vi "Phasor Weber 2-component Calculation.vi"(0 "Phasor 1 (g, s)":T1, 5 "Harmonic Order 1":i32, 7 "Phasor 2 (g, s)":T1, 9 "Harmonic Order 2":i32, 11 "Error In":errorcluster) -> (4 "Reduced Lifetime 1":dbl, 6 "Fraction 1":dbl, 8 "Reduced Lifetime 2":dbl, 10 "Fraction 2":dbl, 15 "Error Out":errorcluster)   [LabVIEW 2021, in "Phasor.lvlib"]
uses:
  Phasor (g, s).ctl
  Phasor.lvlib
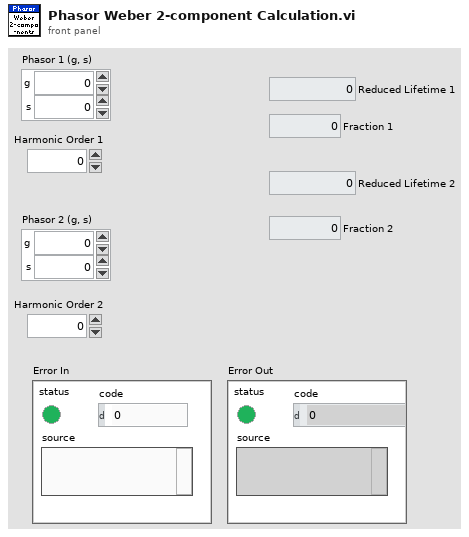
[diagram p1: front panel]
types:
  T1 = typedef "Phasor.lvlib/Phasor (g, s).ctl" = cluster{"g":dbl, "s":dbl}
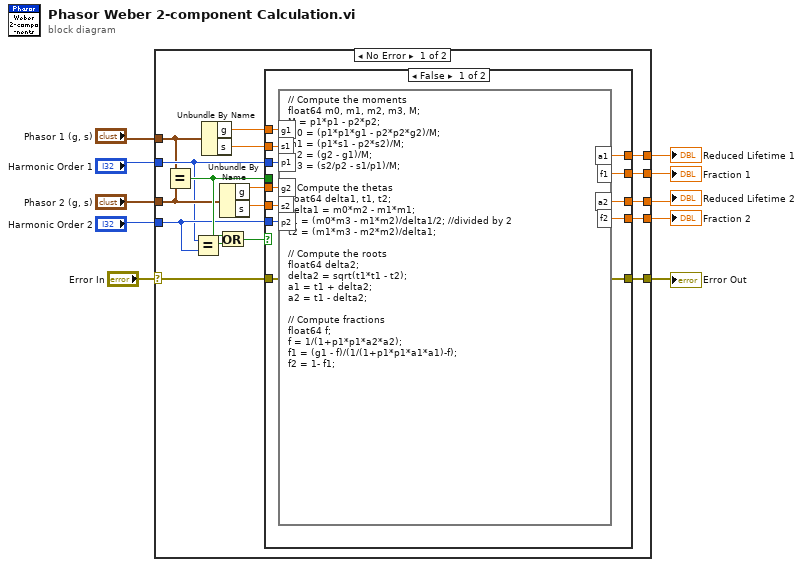
[diagram p0: block diagram]
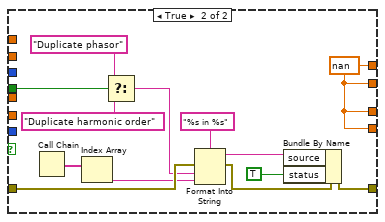
[diagram p2: hidden frame]
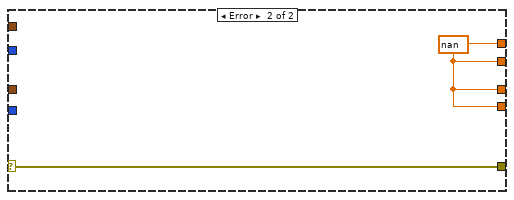
[diagram p3: hidden frame]
diagram:
  n1 = case shown="No Error" "Error In" {
    selector: "Error In" -> [w16 w52]
    tunnel: [w27 w53] -> w2
    tunnel: [w26 w53] -> w1
    tunnel: [w25 w53] -> w4
    tunnel: [w24 w53] -> w3
    tunnel: [w17 w52] -> w9
    tunnel: "Phasor 2 (g, s)" -> [w14 _]
    tunnel: "Harmonic Order 2" -> [w13 _]
    tunnel: "Harmonic Order 1" -> [w12 _]
    tunnel: "Phasor 1 (g, s)" -> [w11 _]
    frame No Error {
      n2 = Equal?(x=w11, y=w14) -> (x = y?=w15:bool)
      n3 = Equal?(x=w12, y=w13) -> (x = y?=w23:bool)
      n4 = Unbundle By Name(w11) -> ("g"=w21:dbl, "s"=w20:dbl)
      n5 = Or(x=w15, y=w23) -> (x .or. y?=w22:bool)
      n6 = Unbundle By Name(w14) -> ("g"=w19:dbl, "s"=w18:dbl)
      n7 = case shown="False" w22 {
        tunnel: [w38 w51] -> w27
        tunnel: [w37 w51] -> w26
        tunnel: [w36 w51] -> w25
        tunnel: [w35 w51] -> w24
        tunnel: w12 -> [w34 _]
        tunnel: w13 -> [w33 _]
        tunnel: w21 -> [w32 _]
        tunnel: w20 -> [w31 _]
        tunnel: w19 -> [w30 _]
        tunnel: w18 -> [w29 _]
        tunnel: [w28 w50] -> w17
        tunnel: w16 -> [w28 w45]
        tunnel: w15 -> [_ w47]
        frame False {
          n8 = formula code="// Compute the moments\nfloat64 m0, m1, m2, m3, M;\nM = p1*p1 - p2*p2;\nm0 = (p1*p1*g1 - p2*p2*g2)/M;\nm1 = (p1*s1 - p2*s2)/M;\nm2 = (g2 - g1)/M;\nm3 = (s2/p2 - s1/p1)/M;\n\n// Compute the thetas\nfloat64 delta1, t1, t2;\ndelta1 = m0*m2 - m1*m1;\nt1 = (m0*m3 - m1*m2)/delta1/2; //divided by 2\nt2 = (m1*m3 - m2*m2)/delta1;\n\n// Compute the roots\nfloat64 delta2;\ndelta2 = sqrt(t1*t1 - t2);\na1 = t1 + delta2;\na2 = t1 - delta2;\n\n// Compute fractions\nfloat64 f;\nf = 1/(1+p1*p1*a2*a2);\nf1 = (g1 - f)/(1/(1+p1*p1*a1*a1)-f);\nf2 = 1- f1;"("g1"=w32, "s1"=w31, "p1"=w34, "g2"=w30, "s2"=w29, "p2"=w33) -> ("a1"=w38:dbl, "f1"=w37:dbl, "a2"=w36:dbl, "f2"=w35:dbl)
        }
        frame True {
          w51 = nan ("a1")
          n9 = Call Chain() -> (call chain=w48:string[])
          n10 = Index Array(array=w48) -> (element=w42:string)  [unwired: 1 in]
          n11 = Select(t="Duplicate phasor" ("format string"), s=w47, f="Duplicate harmonic order" ("format string")) -> (s? t:f=w41:string)
          n12 = Format Into String(format string="%s in %s", error in=w45, w41, w42) -> (resulting string=w46:string, error out=w44:errorcluster)  [unwired: 1 in]
          n13 = Bundle By Name(cluster=w44, "source"=w46, "status"=TRUE) -> (w50:errorcluster)
        }
      }
    }
    frame Error {
      w53 = nan ("a1")
    }
  }
  "Error Out" <- w9
  "Reduced Lifetime 1" <- w2
  "Fraction 1" <- w1
  "Fraction 2" <- w3
  "Reduced Lifetime 2" <- w4
